vi "Set SCIP Mode.vi"(8 "error in (no error)":errorcluster, 10 "Protocol (2: SCIP 2.0)":u32(ring)=2 items=["Convert to Latest", "SCIP 1.1", "SCIP 2.0"], 11 "VISA resource name":refnum<visa-resource-name>) -> (0 "error out":errorcluster, 3 "VISA resource name out":refnum<visa-resource-name>)   [LabVIEW 2011, in "Hokuyo URG Series.lvlib"]
doc: "Sets a SCIP 1.1 instrument to use the SCIP 2.0 protocol. Not all instruments or firmware revisions support this call. Refer to the instrument manual for more informaiton. This VI is called from the initialization VI and should generally not be called on its own."
uses:
  Hokuyo URG Series.lvlib
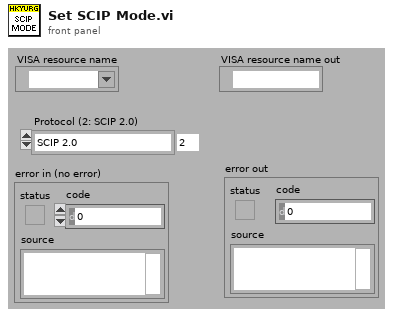
[diagram p1: front panel]
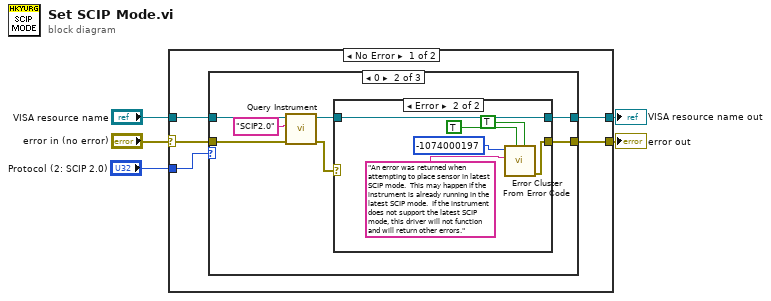
[diagram p0: block diagram]
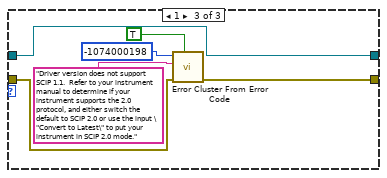
[diagram p4: hidden frame]
diagram:
  n1 = case shown="No Error" "error in (no error)" {
    selector: "error in (no error)" -> [w6 w34]
    tunnel: [w10 w34] -> w5
    tunnel: [w9 w35] -> w4
    tunnel: "VISA resource name" -> [w8 w35]
    tunnel: "Protocol (2: SCIP 2.0)" -> [w7 _]
    frame No Error {
      n2 = case shown="0" w7 {
        tunnel: w8 -> [w12 w18 w32]
        tunnel: [w12 w14 w32] -> w9
        tunnel: w6 -> [w11 w17 w29]
        tunnel: [w11 w13 w33] -> w10
        frame 2, Default {
        }
        frame 0 {
          n3 = call "Query Instrument.vi"("error in"=w17, "Command"="SCIP2.0" ("Change to SCIP 2.0"), "VISA Resource Name"=w18) -> ("error out"=w16:errorcluster, "VISA Resource Name Out"=w15:refnum<visa-resource-name>)  [unwired: 6 in, 1 out]
          n4 = case shown="Error" w16 {
            selector: w16 -> [w20 _]
            tunnel: w15 -> [w21 w24]
            tunnel: [w21 w24] -> w14
            tunnel: [w20 w22] -> w13
            frame No Error {
            }
            frame Error {
              n5 = call <vilib>:"Error Cluster From Error Code.vi"("is warning? (False)"=TRUE, "show call chain? (False)"=TRUE, "error message (\"\")"="An error was returned when attempting to place sensor in latest SCIP mode.  This may happen if the instrument is already running in the latest SCIP mode.  If the instrument does not support the latest SCIP mode, this driver will not function and will return other errors." ("error message (\"\")"), "error code (0)"=-1074000197) -> ("error out"=w22:errorcluster)  [unwired: 5 in]
            }
          }
        }
        frame 1 {
          n6 = call <vilib>:"Error Cluster From Error Code.vi"("show call chain? (False)"=TRUE, "error in (no error)"=w29, "error message (\"\")"="Driver version does not support SCIP 1.1.  Refer to your instrument manual to determine if your instrument supports the 2.0 protocol, and either switch the default to SCIP 2.0 or use the input \"Convert to Latest\" to put your instrument in SCIP 2.0 mode." ("error message (\"\")"), "error code (0)"=-1074000198) -> ("error out"=w33:errorcluster)  [unwired: 5 in]
        }
      }
    }
    frame Error {
    }
  }
  "error out" <- w5
  "VISA resource name out" <- w4
